vi "Insert Error.vi"(8 "Message":string, 9 "Insert (T)":bool=TRUE, 10 "Code (5000)":i32=5000, 11 "Error In":errorcluster) -> (3 "Error Out":errorcluster)   [LabVIEW 2017, in "Configit.lvlib"]
uses:
  Configit.lvlib
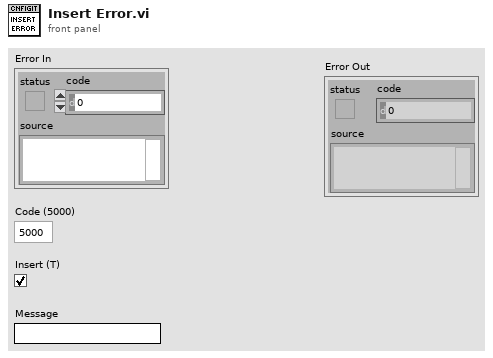
[diagram p1: front panel]
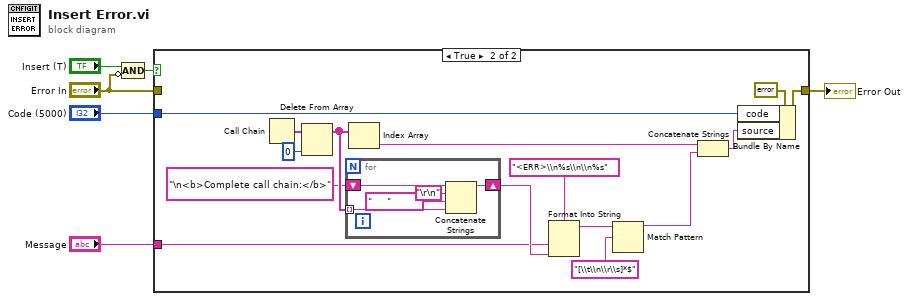
[diagram p0: block diagram]
diagram:
  n1 = Compound Arithmetic op=AND("Insert (T)", invert "Error In") -> (w1:bool)
  n2 = case shown="True" w1 {
    tunnel: [w7 w22] -> w2
    tunnel: "Code (5000)" -> [_ w8]
    tunnel: "Error In" -> [w7 _]
    tunnel: "Message" -> [_ w16]
    frame False {
    }
    frame True {
      n3 = Call Chain() -> (call chain=w19:string[])
      n4 = Delete From Array(array=w19, index=0) -> (array with subset deleted=w11:string[])  [unwired: 1 in, 1 out]
      n5 = for {
        tunnel: w11 -> [w24] mode=indexing
        shift-right: [w27] -> w17
        shift-left: "\n<b>Complete call chain:</b>" ("call chain header") -> [w25]
        n6 = Concatenate Strings(w25, "\r\n", "     ", w24) -> (w27:string)
      }
      n7 = Index Array(array=w11) -> (element=w13:string)  [unwired: 1 in]
      n8 = Format Into String(format string="<ERR>\\n%s\\n\\n%s", w16, w17) -> (resulting string=w14:string)  [unwired: 2 in, 1 out]
      n9 = Match Pattern(string=w14, regular expression="[\\t\\n\\r\\s]*$") -> (before substring=w9:string)  [unwired: 1 in, 3 out]
      n10 = Concatenate Strings(w13, w9) -> (w20:string)
      n11 = Bundle By Name(cluster=errorcluster {"status"=TRUE, "code"=0, "source"=""} ("error out"), "code"=w8, "source"=w20) -> (w22:errorcluster)
    }
  }
  "Error Out" <- w2
